vi "set_config_cluster.vi"(8 "error in (no error)":errorcluster, 10 "config cluster variant":variant, 11 "TrajectoryRK110428Fiber in":refnum<class "TrajectoryRK110428Fiber_Spiral.lvclass">) -> (0 "error out":errorcluster, 3 "TrajectoryRK110428Fiber out":refnum<class "TrajectoryRK110428Fiber_Spiral.lvclass">)   [LabVIEW 2010, in "TrajectoryRK110428Fiber_Spiral.lvclass"]
uses:
  TrajectoryRK110428Fiber_Spiral.lvclass
  TrajectoryRK110428Fiber_Spiral.lvclass/TrajectoryRK110428Fiber_Spiral.ctl
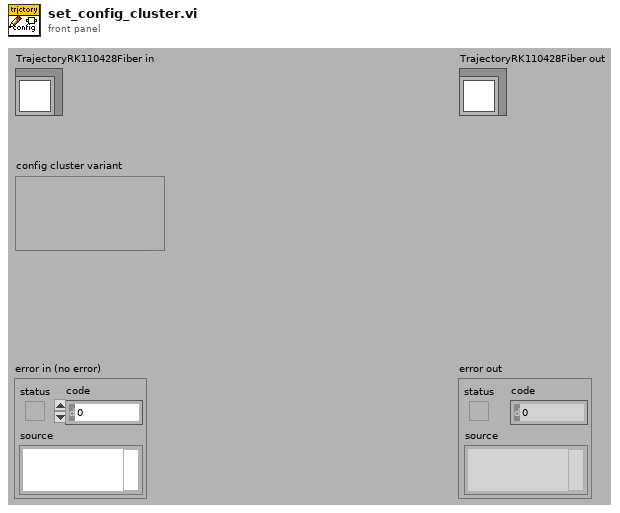
[diagram p1: front panel]
types:
  T1 = typedef "TrajectoryRK110428Fiber.lvclass/config_data_cluster.ctl" = cluster{"FPGAWrapper":T2}
  T2 = typedef "plugin_specification.ctl" = cluster{"class path":string, "configuration":string, "label":string, "settings name":string}
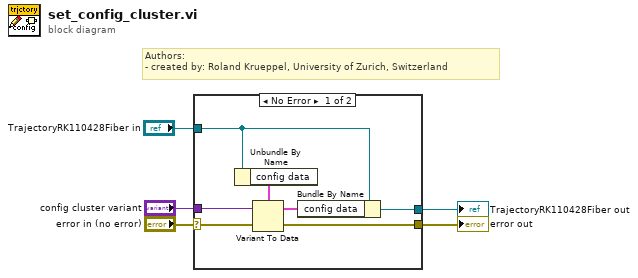
[diagram p0: block diagram]
diagram:
  # "Authors: \n- created by: Roland Krueppel, University of Zurich, Switzerland"
  n1 = case shown="No Error" "error in (no error)" {
    selector: "error in (no error)" -> [w12 w13]
    tunnel: [w11 w13] -> w4
    tunnel: "config cluster variant" -> [w10 _]
    tunnel: "TrajectoryRK110428Fiber in" -> [w8 w14]
    tunnel: [w6 w14] -> w1
    frame No Error {
      n2 = Unbundle By Name(w8) -> ("config data"=w9:T1)
      n3 = Variant To Data(error in=w12, Variant=w10, type=w9) -> (error out=w11:errorcluster, data=w7:T1)
      n4 = Bundle By Name(cluster=w8, "config data"=w7) -> (w6:refnum<class "TrajectoryRK110428Fiber_Spiral.lvclass">)
    }
    frame Error {
    }
  }
  "error out" <- w4
  "TrajectoryRK110428Fiber out" <- w1
